vi "produce last time data.vi"(11 "Array":string[][](array[string])) -> (3 "String":string)   [LabVIEW 2018]
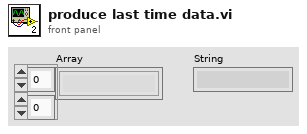
[diagram p1: front panel]
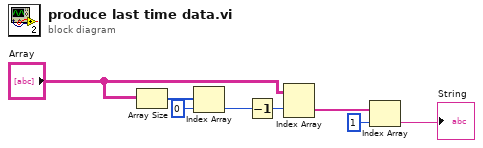
[diagram p0: block diagram]
diagram:
  n1 = Array Size(array="Array") -> (size(s)=w4:i32[])
  n2 = Index Array(array=w4, index=0) -> (element=w5:i32)
  n3 = Decrement(x=w5) -> (x-1=w1:i32)
  n4 = Index Array(array="Array", index (row)=w1) -> (element=w7:string[])  [unwired: 1 in]
  n5 = Index Array(array=w7, index=1) -> (element=→"String":string)
